vi "Read input_.vi"(8 "error in":errorcluster, 11 "DecideProjectFeatures in":refnum<class "UserTBModuleDecideFeatures.lvclass">) -> (0 "error out":errorcluster, 2 "input?":bool, 3 "DecideProjectFeatures out":refnum<class "UserTBModuleDecideFeatures.lvclass">)   [LabVIEW 2013, in "UserTBModuleDecideFeatures.lvclass"]
uses:
  UserTBModuleDecideFeatures.lvclass
  UserTBModuleDecideFeatures.lvclass/UserTBModuleDecideFeatures.ctl
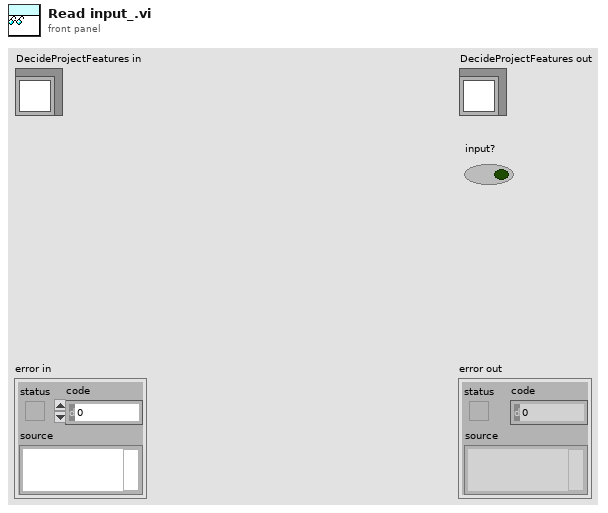
[diagram p1: front panel]
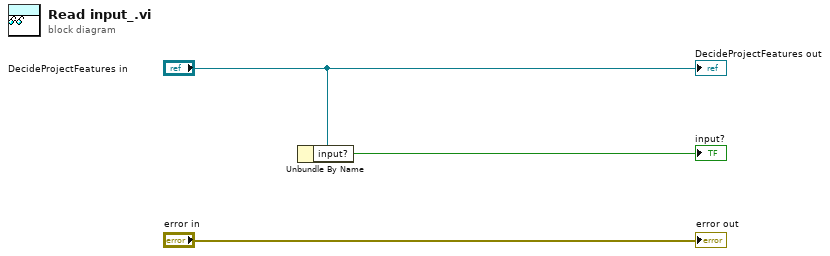
[diagram p0: block diagram]
diagram:
  n1 = Unbundle By Name("DecideProjectFeatures in") -> ("input?"=→"input?":bool)
  "error out" <- "error in"
  "DecideProjectFeatures out" <- "DecideProjectFeatures in"
